vi "PosStrikerAfterPass.vi"(10 "IA Input":T1={"our_robots"=[], "enemy_robots"=[], "balls"=[], "geometry"={"line_width"=0, "field_length"=0, "field_width"=0, "boundary_width"=0, "referee_width"=0, "goal_width"=0, "goal_depth"=0, "goal_wall_width"=0, "center_circle_radius"=0, "defense_radius"=0, "defense_stretch"=0, "free_kick_from_defense_dist"=0, "penalty_spot_from_field_line_dist"=0, "penalty_line_from_spot_dist"=0}, "IA Judge"={"stage"="", "command"="", "our_goalie_id"=0.0, "enemy_goalie_id"=0.0, "command enum"=enum."Halt", "Time"=enum."Azul"}, "Received Timestamp"=timestamp(0 s since 1904-01-01), "Events"={"Touch"=FALSE, "Ball out"=FALSE, "id touch"=0.0, "Ball out of \nVision"=FALSE, "Ball inside \nGoalie area"=FALSE, "Robot not responding"=FALSE, "Robots responding status"=[1.0, 1.0, 1.0, 1.0, 1.0, 1.0], "Enemy Ball \nPossession"=FALSE, "Pass State"=FALSE, "id end of pass"=0.0, "Kick"=FALSE, "Id ini Possession"=0.0, "Ball Possesion"=FALSE, "Id Possesion"=0.0, "Direct Kick"=FALSE, "2nd Strk Ativo"=FALSE}}, 11 "Robot in":T2={"id"=5, "function"=enum."Attacker", "x"=-1842.5054931640625, "y"=520.60986328125, "orientation"=-2.7555055618286133, "v_tangent"=0.0, "v_normal"=0.0, "v_ang"=0.0, "kick_x"=0.0, "kick_z"=0.0, "dribble"=FALSE, "Timestamp"=timestamp(2082758857.4639893 s since 1904-01-01), "estimatives"={"est_v_tangent"=0.0, "est_v_normal"=0.0, "est_vx"=0.0, "est_vy"=0.0, "Pos Robot Est"=[]}, "dest_x_kick"=0.0, "dest_y_kick"=0.0, "Gap Coord"=[], "States"=enum."GoToTangent", "Path "=[], "Path  Smooth"=[], "Dest"=[]}) -> (3 "Robot out":T2={"id"=5, "function"=enum."Attacker", "x"=-1842.5054931640625, "y"=520.60986328125, "orientation"=-2.7555055618286133, "v_tangent"=-0.08361641967936218, "v_normal"=-0.20513016702014014, "v_ang"=0.24456003022714357, "kick_x"=0.0, "kick_z"=0.0, "dribble"=FALSE, "Timestamp"=timestamp(2082758857.4639893 s since 1904-01-01), "estimatives"={"est_v_tangent"=0.0, "est_v_normal"=0.0, "est_vx"=0.0, "est_vy"=0.0, "Pos Robot Est"=[]}, "dest_x_kick"=0.0, "dest_y_kick"=0.0, "Gap Coord"=[], "States"=enum."GoToTangent", "Path "=[], "Path  Smooth"=[], "Dest"=[]})   [LabVIEW 2017]
uses:
  Core/AI Robot.ctl
  Functions Enum.ctl
  AttackerStates.ctl
  Path Planning/RRT/PathDests.ctl
  Path Planning/RRT/PathDest.ctl
  Core/AI Input.ctl
  Core/AI Ball.ctl
  Core/Field Size.ctl
  Core/AI Judge.ctl
  Command Enum.ctl
  Util/Events/Events.ctl
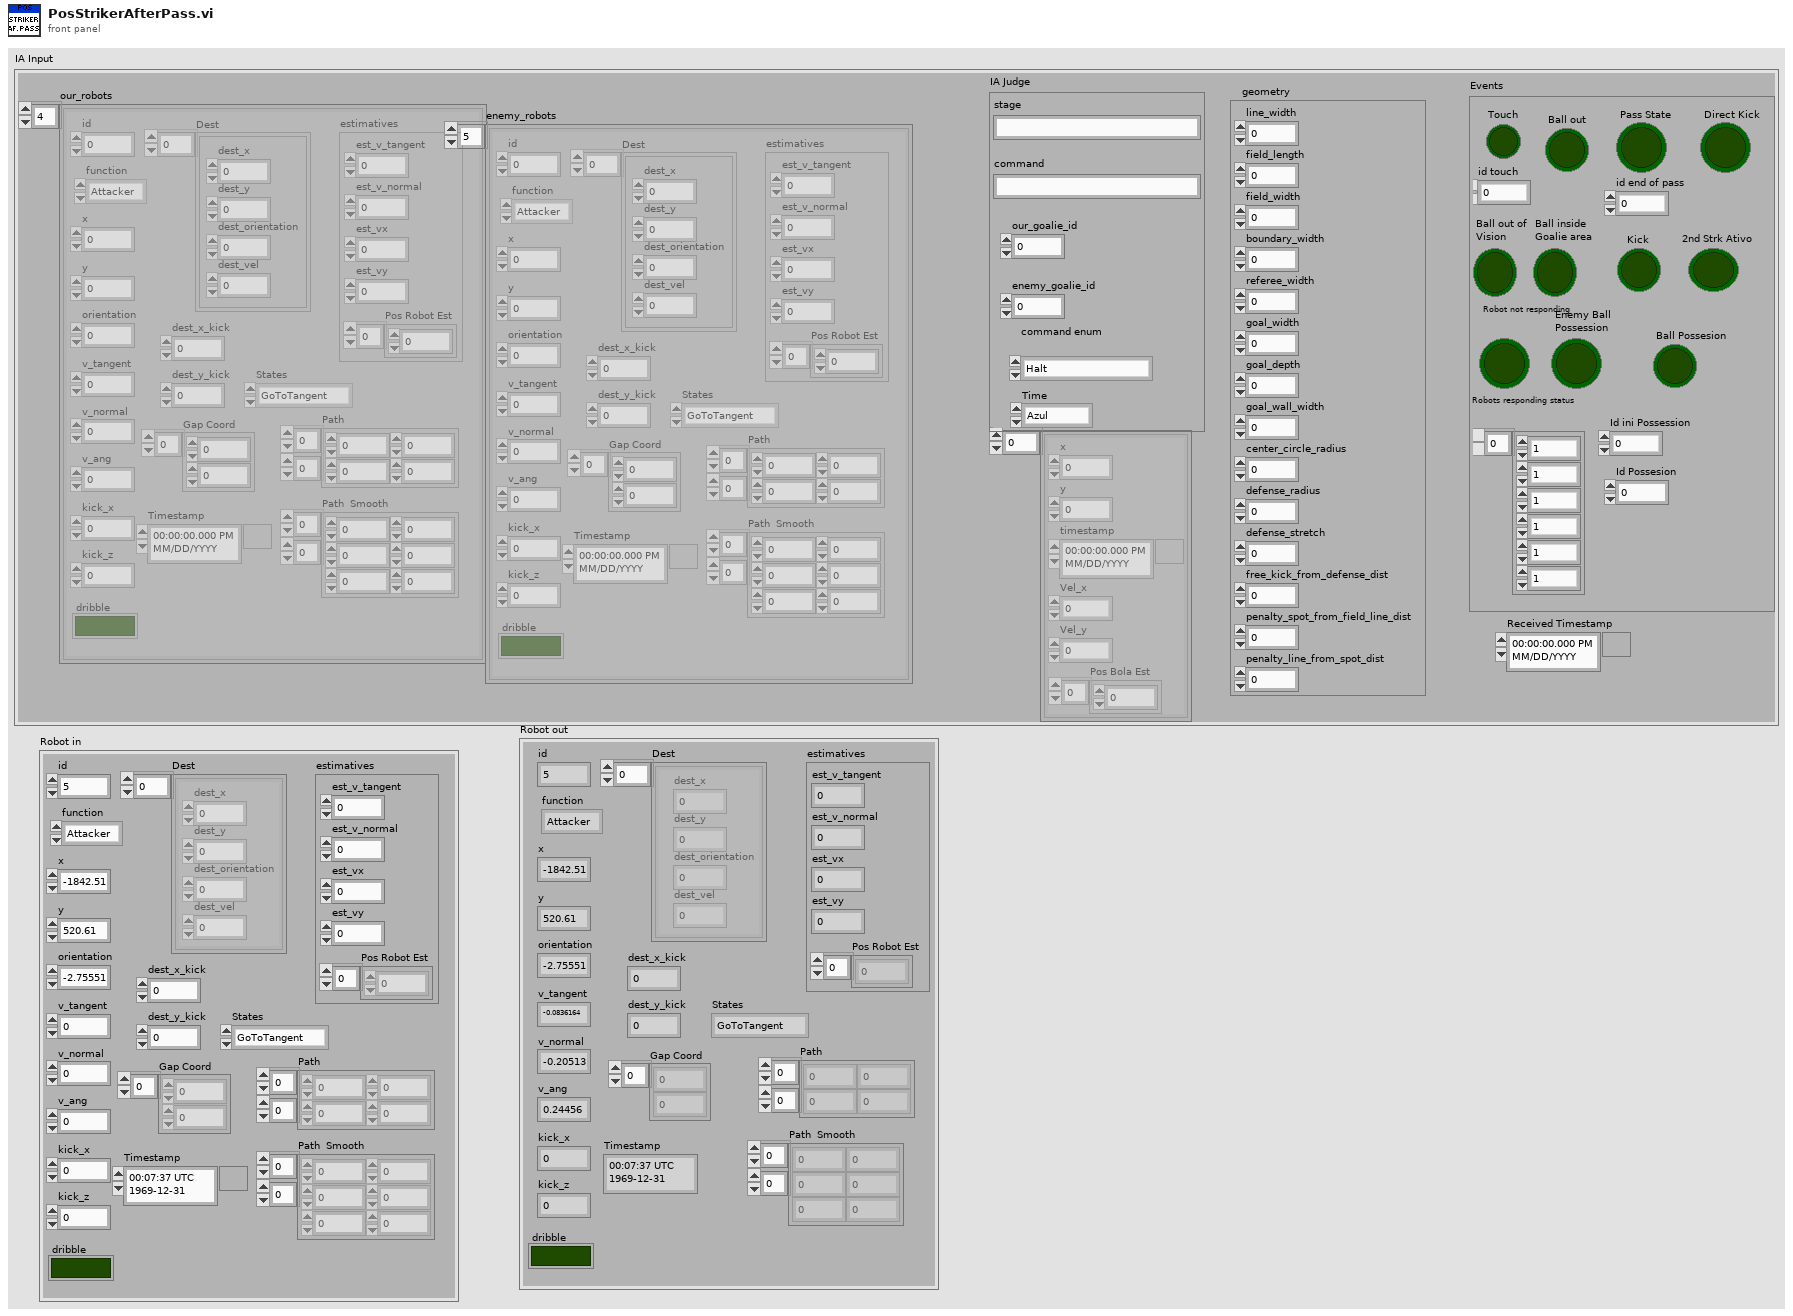
[diagram p1: front panel]
types:
  T1 = typedef "AI Input.ctl" = cluster{"our_robots":T2[], "enemy_robots":T2[], "balls":T7[], "geometry":T8, "IA Judge":T9, "Received Timestamp":timestamp, "Events":T11}
  T2 = typedef "AI Robot.ctl" = cluster{"id":u32, "function":T3, "x":dbl, "y":dbl, "orientation":dbl, "v_tangent":dbl, "v_normal":dbl, "v_ang":dbl, "kick_x":dbl, "kick_z":dbl, "dribble":bool, "Timestamp":timestamp, "estimatives":cluster{"est_v_tangent":dbl, "est_v_normal":dbl, "est_vx":dbl, "est_vy":dbl, "Pos Robot Est":dbl[]}, "dest_x_kick":dbl, "dest_y_kick":dbl, "Gap Coord":dbl[], "States":T4, "Path ":dbl[][], "Path  Smooth":dbl[][], "Dest":T5}
  T3 = typedef "Functions Enum.ctl" = enum16{"2nd Striker", "Attacker", "Goalie", "Defender", "Striker", "Goto 0", "Dummy", "Kicker", "ZigZag 0", "ZigZag 1", "ZigZag 2", "ZigZag 3", "ZigZag 4", "ZigZag 5", "ZigZag 6", "ZigZag 7", "ZigZag 8", ""}
  T4 = typedef "AttackerStates.ctl" = enum16{"Pass", "GoToTangent", "BallGetting", "GoToKick", ""}
  T5 = typedef "PathDests.ctl" = T6[]
  T6 = typedef "PathDest.ctl" = cluster{"dest_x":dbl, "dest_y":dbl, "dest_orientation":dbl, "dest_vel":dbl}
  T7 = typedef "AI Ball.ctl" = cluster{"x":dbl, "y":dbl, "timestamp":timestamp, "Vel_x":dbl, "Vel_y":dbl, "Pos Bola Est":dbl[]}
  T8 = typedef "Field Size.ctl" = cluster{"line_width":u32, "field_length":u32, "field_width":u32, "boundary_width":u32, "referee_width":u32, "goal_width":u32, "goal_depth":u32, "goal_wall_width":u32, "center_circle_radius":u32, "defense_radius":u32, "defense_stretch":u32, "free_kick_from_defense_dist":u32, "penalty_spot_from_field_line_dist":u32, "penalty_line_from_spot_dist":u32}
  T9 = typedef "AI Judge.ctl" = cluster{"stage":string, "command":string, "our_goalie_id":dbl, "enemy_goalie_id":dbl, "command enum":T10, "Time":enum16{"Azul", "Amarelo"}}
  T10 = typedef "Command Enum.ctl" = enum16{"Halt", "Stop", "Force Start", "PKA Normal Start", "Prepare Kickoff Ally", "PKE Normal Start", "Prepare Kickoff Enemy", "Prepare Penalty Ally", "PPA Normal Start", "Prepare Penalty Enemy", "PPE Normal Start", "Direct Free Enemy", "Direct Free Ally", "Indirect Free Enemy", "Indirect Free Ally", "Timeout Enemy", "Timeout Ally", "Goal Enemy", "Goal Ally", "Ball Placement Enemy", "Ball Placement Ally", "Normal Half Time", "Extra Time Break", "Extra Half Time", "None", "Post Game"}
  T11 = typedef "Events.ctl" = cluster{"Touch":bool, "Ball out":bool, "id touch":dbl, "Ball out of \nVision":bool, "Ball inside \nGoalie area":bool, "Robot not responding":bool, "Robots responding status":dbl[], "Enemy Ball \nPossession":bool, "Pass State":bool, "id end of pass":dbl, "Kick":bool, "Id ini Possession":dbl, "Ball Possesion":bool, "Id Possesion":dbl, "Direct Kick":bool, "2nd Strk Ativo":bool}
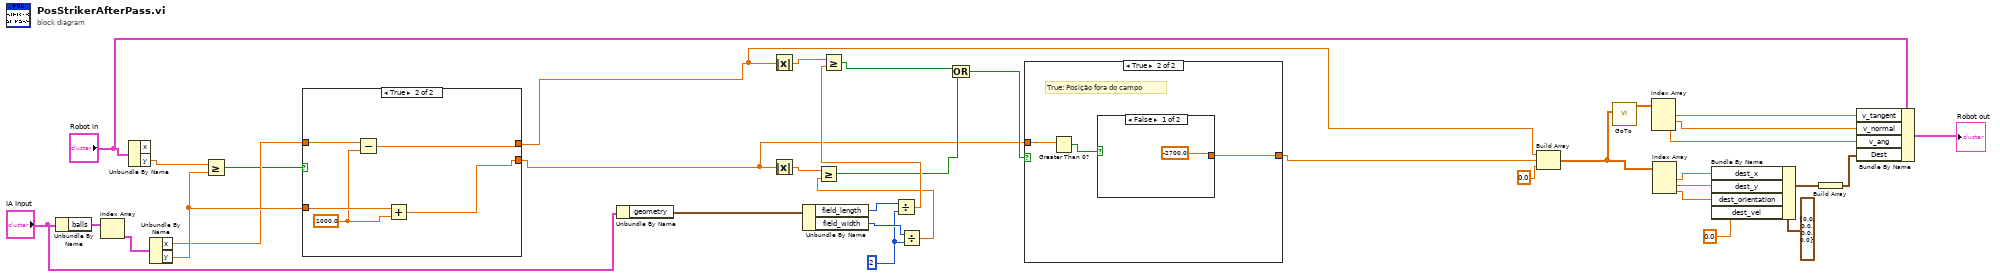
[diagram p0: block diagram]
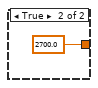
[diagram p3: hidden frame]
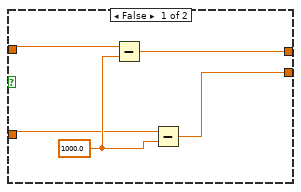
[diagram p4: hidden frame]
diagram:
  w5 = u32 2 ("field_length")
  n1 = Unbundle By Name("IA Input") -> ("balls"=w36:T7[])
  n2 = Index Array(array=w36) -> (element=w35:T7)  [unwired: 1 in]
  n3 = Unbundle By Name("Robot in") -> ("y"=w34:dbl)  [unwired: 1 out]
  n4 = Unbundle By Name(w35) -> ("x"=w32:dbl, "y"=w33:dbl)
  n5 = Greater Or Equal?(x=w34, y=w33) -> (x >= y?=w31:bool)
  n6 = case shown="True" w31 {
    tunnel: w33 -> [w40 w46]
    tunnel: w32 -> [w39 w45]
    tunnel: [w38 w43] -> w3
    tunnel: [w37 w42] -> w4
    frame False {
      w41 = 1000.0 ("y")
      n7 = Subtract(x=w39, y=w41) -> (x-y=w38:dbl)
      n8 = Subtract(x=w40, y=w41) -> (x-y=w37:dbl)
    }
    frame True {
      w44 = 1000.0 ("y")
      n9 = Subtract(x=w45, y=w44) -> (x-y=w43:dbl)
      n10 = Add(x=w46, y=w44) -> (x+y=w42:dbl)
    }
  }
  n11 = Unbundle By Name("IA Input") -> ("geometry"=w15:T8)
  n12 = Absolute Value(x=w3) -> (abs(x)=w7:dbl)
  n13 = Absolute Value(x=w4) -> (abs(x)=w11:dbl)
  n14 = Unbundle By Name(w15) -> ("field_length"=w14:u32, "field_width"=w13:u32)
  n15 = Divide(x=w14, y=w5) -> (x/y=w12:dbl)
  n16 = Greater Or Equal?(x=w7, y=w12) -> (x >= y?=w8:bool)
  n17 = Divide(x=w13, y=w5) -> (x/y=w10:dbl)
  n18 = Greater Or Equal?(x=w11, y=w10) -> (x >= y?=w9:bool)
  n19 = Or(x=w8, y=w9) -> (x .or. y?=w6:bool)
  n20 = case shown="True" w6 {
    tunnel: w4 -> [w47 w50]
    tunnel: [w47 w48] -> w2
    frame False {
      # "True: Posição detnro do campo"
    }
    frame True {
      # "True: Posição fora do campo"
      n21 = Greater Than 0?(x=w50) -> (x > 0?=w49:bool)
      n22 = case shown="False" w49 {
        tunnel: [-2700.0 2700.0] -> w48
        frame False {
        }
        frame True {
        }
      }
    }
  }
  n23 = Build Array(w3, w2, 0.0 ("element")) -> (w16:dbl[])
  n24 = call "GoTo.vi"("Target"=w16) -> ("Output\nVelocity"=w30:dbl[])  [unwired: 9 in, 1 out]
  n25 = Index Array(array=w30) -> (element #1=w29:dbl, element #2=w28:dbl, element #3=w27:dbl)  [unwired: 3 in]
  n26 = Index Array(array=w16) -> (element #1=w22:dbl, element #2=w21:dbl, element #3=w20:dbl)  [unwired: 3 in]
  n27 = Bundle By Name(cluster=T6 {"dest_x"=0.0, "dest_y"=0.0, "dest_orientation"=0.0, "dest_vel"=0.0} ("Dest"), "dest_x"=w22, "dest_y"=w21, "dest_orientation"=w20, "dest_vel"=0.0) -> (w25:T6)
  n28 = Build Array(w25) -> (w23:T6[])
  n29 = Bundle By Name(cluster="Robot in", "v_tangent"=w29, "v_normal"=w28, "v_ang"=w27, "Dest"=w23) -> (→"Robot out":T2)
